vi "Generate Printf Event.vi"(8 "error in (no error)":errorcluster, 9 "Verbose Level":i32, 10 "Printf Message":refnum<class "LV_Printf Msg.lvclass">) -> (0 "error out":errorcluster)   [LabVIEW 2013, in "SET_Printf.lvlib" / "LV_Printf Core.lvclass"]
uses:
  LV_Printf Core.lvclass
  Messages/General/LV_Printf Msg.lvclass
  LV_Printf Core.lvclass/LV_Printf Core.ctl
panel:
  # "Generates a printf event if specified verbose level is greater than or equal to the\nconfigured verbose level."
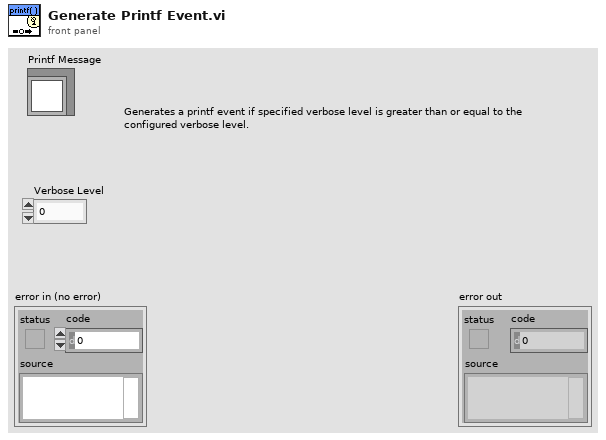
[diagram p1: front panel]
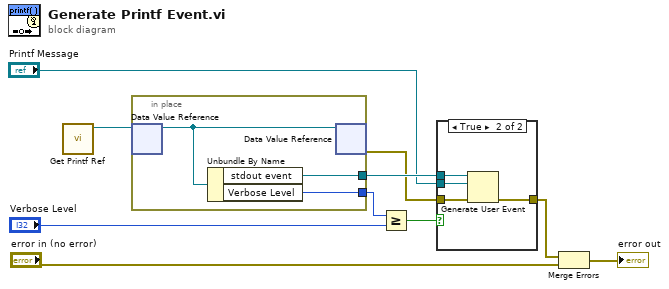
[diagram p0: block diagram]
diagram:
  n1 = call "Get Printf Ref.vi"() -> ("Printf DVR"=w10:refnum<data-value>)  [unwired: 11 in]
  n2 = in-place {
    in-place-border: [w13] -> w7
    in-place-border: [w12] -> w3
    n3 = in-place-dvr #1(w10) -> (w11:refnum<class "LV_Printf Core.lvclass">)  [unwired: 1 out]
    n4 = Unbundle By Name(w11) -> ("stdout event"=w13:refnum<user-event>, "Verbose Level"=w12:i32)
    n5 = in-place-dvr #1(w11) -> (w6:errorcluster)  [unwired: 1 out]
  }
  n6 = Greater Or Equal?(x=w3, y="Verbose Level") -> (x >= y?=w1:bool)
  n7 = case shown="True" w1 {
    tunnel: w7 -> [_ w18]
    tunnel: w6 -> [w14 w17]
    tunnel: "Printf Message" -> [_ w16]
    tunnel: [w14 w15] -> w4
    frame False {
    }
    frame True {
      n8 = Generate User Event(user event=w18, event data cluster=w16, error in=w17) -> (error out=w15:errorcluster)  [unwired: 1 in, 1 out]
    }
  }
  n9 = Merge Errors(w4, "error in (no error)") -> (→"error out":errorcluster)
